vi "Filter_Indices.vi"(9 "Filter Range":i32=4, 10 "Array to Filter":i32[](array[numeric])) -> (0 "Ignored For":i32[](array[numeric]), 1 "Ignore and Remove":i32[](array[numeric]), 2 "Cleaned Array":i32[](array[numeric]))   [LabVIEW 2016]
panel:
  out "Array":i32
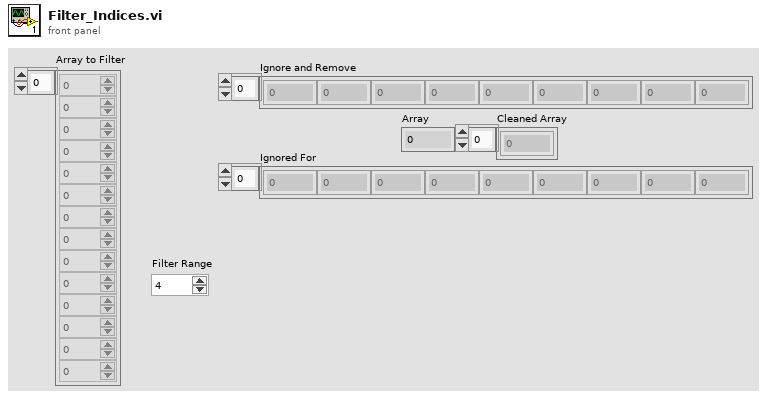
[diagram p1: front panel]
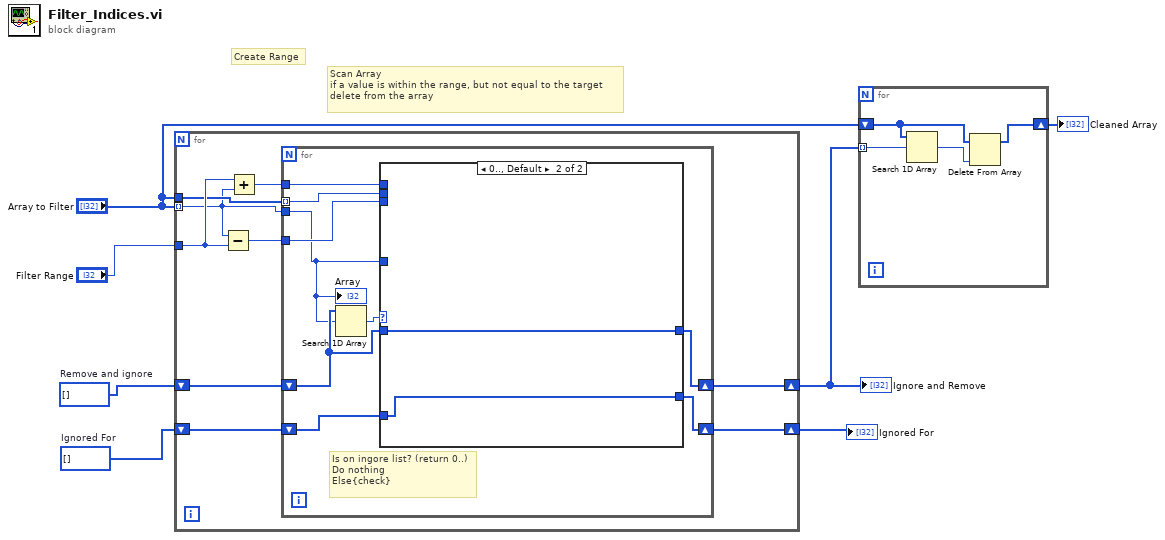
[diagram p0: block diagram]
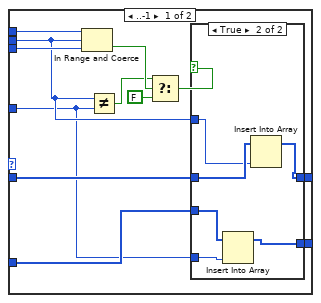
[diagram p2: hidden frame]
diagram:
  w2 = i32[] []  # Ignored For
  w6 = i32[] []  # Remove and ignore
  # "Scan Array\nif a value is within the range, but not equal to the target\ndelete from the array"
  # "Create Range"
  n1 = for {
    tunnel: "Array to Filter" -> [w12] mode=indexing
    tunnel: "Filter Range" -> [w16]
    tunnel: "Array to Filter" -> [w13]
    shift-right: [w11] -> w4
    shift-left: w6 -> [w10]
    shift-right: [w8] -> w1
    shift-left: w2 -> [w9]
    n2 = Subtract(x=w12, y=w16) -> (x-y=w14:i32)
    n3 = Add(x=w16, y=w12) -> (x+y=w15:i32)
    n4 = for {
      tunnel: w15 -> [w25]
      tunnel: w14 -> [w24]
      tunnel: w13 -> [w23] mode=indexing
      tunnel: w12 -> [w19]
      shift-right: [w20] -> w11
      shift-left: w10 -> [w21]
      shift-right: [w18] -> w8
      shift-left: w9 -> [w17]
      # "Is on ingore list? (return 0..)\nDo nothing\nElse{check}"
      n5 = Search 1D Array(1D array=w21, element=w19) -> (index of element=w22:i32)  [unwired: 1 in]
      n6 = case shown="0.., Default" w22 {
        tunnel: w25 -> [w37 _]
        tunnel: w24 -> [w36 _]
        tunnel: w19 -> [w26 _]
        tunnel: w23 -> [w31 _]
        tunnel: w21 -> [w29 w47]
        tunnel: [w30 w47] -> w20
        tunnel: [w28 w46] -> w18
        tunnel: w17 -> [w27 w46]
        frame ..-1 {
          n7 = In Range and Coerce(upper limit=w37, x=w31, lower limit=w36) -> (In Range?=w35:bool)  [unwired: 1 out]
          n8 = Not Equal?(x=w31, y=w26) -> (x != y?=w34:bool)
          n9 = Select(t=w34, s=w35, f=FALSE) -> (s? t:f=w33:bool)
          n10 = case shown="True" w33 {
            tunnel: w31 -> [_ w43]
            tunnel: [w39 w44] -> w30
            tunnel: w29 -> [w39 w45]
            tunnel: [w38 w41] -> w28
            tunnel: w27 -> [w38 w42]
            tunnel: w26 -> [_ w40]
            frame False {
            }
            frame True {
              n11 = Insert Into Array(array=w42, new element=w40) -> (w41:i32[])  [unwired: 1 in]
              n12 = Insert Into Array(array=w45, new element=w43) -> (w44:i32[])  [unwired: 1 in]
            }
          }
        }
        frame 0.., Default {
        }
      }
      "Array" <- w19
    }
  }
  "Ignore and Remove" <- w4
  "Ignored For" <- w1
  n13 = for {
    tunnel: w4 -> [w51] mode=indexing
    shift-right: [w48] -> w3
    shift-left: "Array to Filter" -> [w49]
    n14 = Search 1D Array(1D array=w49, element=w51) -> (index of element=w50:i32)  [unwired: 1 in]
    n15 = Delete From Array(array=w49, index=w50) -> (array with subset deleted=w48:i32[])  [unwired: 1 in, 1 out]
  }
  "Cleaned Array" <- w3
